vi "Funktionen Schalten AutoKal alt.vi"() -> (3 "AutoKal":T1)   [LabVIEW 2020, in "Allgemein.lvlib"]
uses:
  Allgemein.lvlib
  FGV Analysator aktiv.ctl
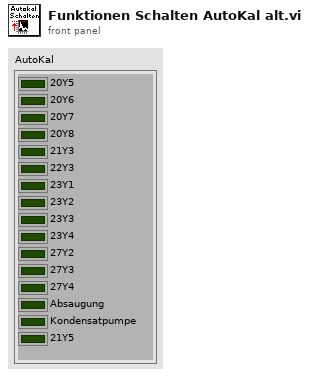
[diagram p1: front panel]
types:
  T1 = cluster{"20Y5":bool, "20Y6":bool, "20Y7":bool, "20Y8":bool, "21Y3":bool, "22Y3":bool, "23Y1":bool, "23Y2":bool, "23Y3":bool, "23Y4":bool, "27Y2":bool, "27Y3":bool, "27Y4":bool, "Absaugung":bool, "Kondensatpumpe":bool, "21Y5":bool}
  T2 = typedef "Allgemein.lvlib/FGV Analysator aktiv.ctl" = enum16{"lesen", "Analysator", "CG Aufschaltung", "KAL Zustand", "AutaKal GT?"}
  T3 = typedef "Auto Kalibrieren.lvlib/KalibrierZustaende.ctl" = cluster{"FTIR Zustand":u16, "PMA Zustand":u16, "FID CH4 Zustand":u16, "FID THC Zustand":u16, "FID THC CG":u16}
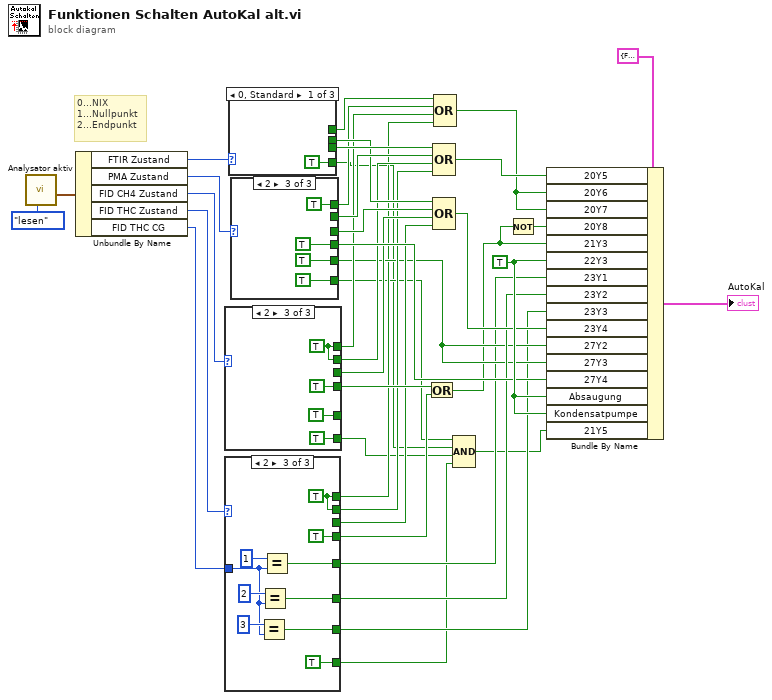
[diagram p0: block diagram]
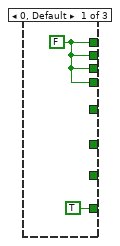
[diagram p2: hidden frame]
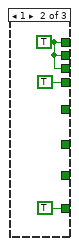
[diagram p3: hidden frame]
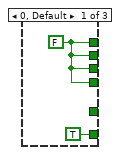
[diagram p4: hidden frame]
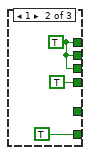
[diagram p5: hidden frame]
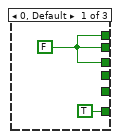
[diagram p6: hidden frame]
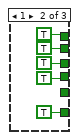
[diagram p7: hidden frame]
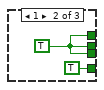
[diagram p8: hidden frame]
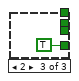
[diagram p9: hidden frame]
diagram:
  w33 = TRUE ("20Y6")
  # "0...NIX\n1...Nullpunkt\n2...Endpunkt"
  n1 = call "Analysator aktiv.vi"("Aktion"=FGV_Analysator_aktiv."lesen") -> ("Kalibrieren"=w37:T3)  [unwired: 7 in, 3 out]
  n2 = Unbundle By Name(w37) -> ("FTIR Zustand"=w36:u16, "PMA Zustand"=w32:u16, "FID CH4 Zustand"=w24:u16, "FID THC Zustand"=w15:u16, "FID THC CG"=w10:u16)
  n3 = case shown="2" w24 {
    tunnel: [w41 w44 w47] -> w22
    tunnel: [w41 w44 w47] -> w21
    tunnel: [w41 w44 _] -> w20
    tunnel: [w41 TRUE ("Zeit abgelaufen?") TRUE ("Zeit abgelaufen?")] -> w23
    tunnel: [_ _ TRUE ("Zeit abgelaufen?")] -> _
    tunnel: [TRUE ("Zeit abgelaufen?") TRUE ("Zeit abgelaufen?") TRUE ("Zeit abgelaufen?")] -> w5
    frame 0, Default {
      w41 = FALSE
    }
    frame 1 {
      w44 = TRUE
    }
    frame 2 {
      w47 = TRUE
    }
  }
  n4 = case shown="2" w15 {
    tunnel: [w50 w53 w62] -> w11
    tunnel: [w50 w53 w62] -> w19
    tunnel: [w50 w53 _] -> w18
    tunnel: [w50 TRUE ("Zeit abgelaufen?") TRUE ("Zeit abgelaufen?")] -> w17
    tunnel: [_ _ w59] -> w16
    tunnel: w10 -> [_ _ w57]
    tunnel: [_ _ w56] -> w9
    tunnel: [_ _ w55] -> w8
    tunnel: [TRUE ("Zeit abgelaufen?") TRUE ("Zeit abgelaufen?") TRUE ("Zeit abgelaufen?")] -> w4
    frame 0, Default {
      w50 = FALSE
    }
    frame 1 {
      w53 = TRUE
    }
    frame 2 {
      w62 = TRUE
      n5 = Equal?(x=u16 3, y=w57) -> (x = y?=w55:bool)
      n6 = Equal?(x=u16 2, y=w57) -> (x = y?=w59:bool)
      n7 = Equal?(x=u16 1, y=w57) -> (x = y?=w56:bool)
    }
  }
  n8 = case shown="0, Standard" w36 {
    tunnel: [_ w66 _] -> w30
    tunnel: [_ w66 _] -> w34
    tunnel: [_ w66 _] -> w27
    tunnel: [TRUE TRUE TRUE] -> w6
    frame 0, Default {
    }
    frame 1 {
      w66 = TRUE
    }
    frame 2 {
    }
  }
  n9 = case shown="2" w32 {
    tunnel: [w69 TRUE _] -> w31
    tunnel: [w69 TRUE _] -> w28
    tunnel: [w69 TRUE TRUE] -> w26
    tunnel: [_ TRUE TRUE] -> w25
    tunnel: [_ _ TRUE] -> w14
    tunnel: [TRUE TRUE TRUE] -> w7
    frame 0, Default {
      w69 = FALSE
    }
    frame 1 {
    }
    frame 2 {
    }
  }
  n10 = Or(x=w23, y=w17) -> (x .or. y?=w13:bool)
  n11 = Compound Arithmetic op=OR(w34, w31, w21, w19) -> (w35:bool)
  n12 = Compound Arithmetic op=OR(w30, w28, w20, w18) -> (w29:bool)
  n13 = Compound Arithmetic op=OR(w27, w26, w22, w11) -> (w2:bool)
  n14 = Compound Arithmetic op=AND ("Mehrfacharithmetik")(w7, w6, w5, w4) -> (w3:bool)
  n15 = Not(x=w13) -> (.not. x?=w12:bool)
  n16 = Bundle By Name(cluster=T1 {"20Y5"=FALSE, "20Y6"=FALSE, "20Y7"=FALSE, "20Y8"=FALSE, "21Y3"=FALSE, "22Y3"=FALSE, "23Y1"=FALSE, "23Y2"=FALSE, "23Y3"=FALSE, "23Y4"=FALSE, "27Y2"=FALSE, "27Y3"=FALSE, "27Y4"=FALSE, "Absaugung"=FALSE, "Kondensatpumpe"=FALSE, "21Y5"=FALSE} ("AutoKal"), "20Y5"=w35, "20Y6"=w2, "20Y7"=w2, "20Y8"=w13, "21Y3"=w12, "22Y3"=w33, "23Y1"=w9, "23Y2"=w16, "23Y3"=w8, "23Y4"=w29, "27Y2"=w14, "27Y3"=w14, "27Y4"=w25, "Absaugung"=w33, "Kondensatpumpe"=w33, "21Y5"=w3) -> (→"AutoKal":T1)
